vi "Eurotherm_write_T.vi"(8 "error in (no error)":errorcluster, 9 "Tª_sp":dbl min=-28.0 max=70.0 step=0.1, 10 "Tª write":bool, 11 "Modbus Master in":refnum<class "Modbus Master.lvclass">) -> (0 "error out":errorcluster, 3 "Modbus Master out":refnum<class "Modbus Master.lvclass">)   [LabVIEW 2021, in "CC_Library.lvlib"]
uses:
  CC_Library.lvlib
  <vilib>/Modbus/master/Modbus Master.lvclass
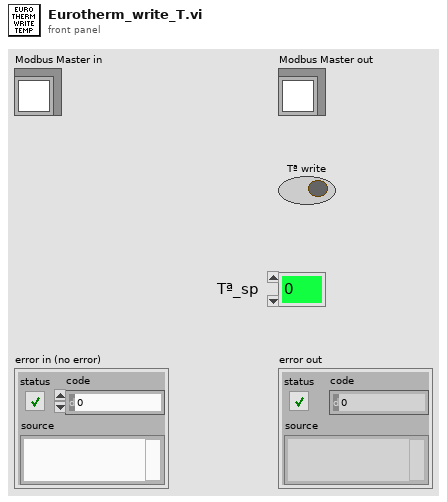
[diagram p1: front panel]
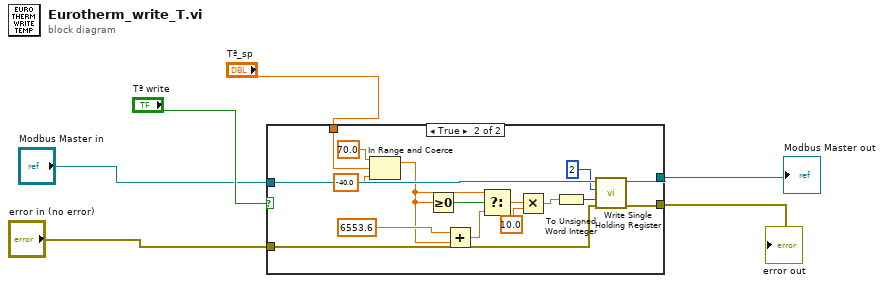
[diagram p0: block diagram]
diagram:
  n1 = case shown="True" "Tª write" {
    tunnel: "Modbus Master in" -> [w8 w24]
    tunnel: "error in (no error)" -> [w7 w23]
    tunnel: [w7 w21] -> w3
    tunnel: [w8 w20] -> w4
    tunnel: "Tª_sp" -> [_ w9]
    frame False {
    }
    frame True {
      n2 = In Range and Coerce(upper limit=70.0, x=w9, lower limit=-40.0) -> (coerced(x)=w10:dbl)  [unwired: 1 out]
      n3 = Greater Or Equal To 0?(x=w10) -> (x >= 0?=w19:bool)
      n4 = Add(x=6553.6, y=w10) -> (x+y=w17:dbl)
      n5 = Select(t=w10, s=w19, f=w17) -> (s? t:f=w13:dbl)
      n6 = Multiply(x=w13, y=10.0) -> (x*y=w14:dbl)
      n7 = To Unsigned Word Integer(number=w14) -> (unsigned 16bit integer=w15:u16)
      n8 = call-dynamic "Write Single Holding Register.vi"("error in (no error)"=w23, "holding register value"=w15, "address"=u16 2, "Modbus master in"=w24) -> ("error out"=w21:errorcluster, "Modbus master out"=w20:refnum<class "Modbus Master.lvclass">)  [unwired: 6 in]
    }
  }
  "Modbus Master out" <- w4
  "error out" <- w3
